vi "Autonomous Independent.vi"   [LabVIEW 2015]
doc: "This VI is called when autonomous begins, and will automatically be terminated when autonomous ends. You can carry out timed or sensor driven robot movement independently without needing to return to the caller."
uses:
  Auton Control.ctl
  <vilib>/Rock Robotics/WPI/Utilities/WPI_GetSetVariantRefNum.vi
  <vilib>/Rock Robotics/Network Tables/NT Read Numeric Array.vi
  <vilib>/Rock Robotics/Network Tables/NT Write Number.vi
  <vilib>/Rock Robotics/Network Tables/NT Write Boolean.vi
  <vilib>/Rock Robotics/Network Tables/NT Write Numeric Array.vi
  navX Library v2/navX Library v2.lvlib
panel:
  # "Be sure to right-click and choose Data Operations>>Make Current Value default if you want to save the array values with the VI"
types:
  T1 = typedef "Auton Control.ctl" = enum16{"Rough Terrain", "Moat", "Ramparts", "Portcullis", "Cheval de Frise", "Rock Wall", "SolenoidControl", "AllStop", "BackOff", "Feeder", "LowBar", "GyroReset", "Shoot", "Scan", "Long Pause", "Short Pause", "Initialize", "Stop", "Straight Forward", "Straight Back", "90 Right", "90 Left", "60 Right", "60 Left"}
  T2 = typedef "WPI_RobotDriveDevRef.ctl" = cluster{"DevStatus":errorcluster, "Motors[]":T3[], "Square Inputs":bool, "Max Output":dbl}
  T3 = typedef "WPI_MotorControlDeviceRef.ctl" = cluster{"DeviceStatus":errorcluster, "Type":T4, "PWM":cluster{"PWM Channel":T5, "DeadBand":T6}, "CAN":cluster{"Device Number":u8, "Control Mode":T7, "Semaphore":T8, "Max Vout":dbl, "TalonSRX Control Mode":T9}, "Invert":bool}
  T4 = typedef "WPI_MotorControlType.ctl" = enum16{"PWM", "CAN", "CANTalonSRX"}
  T5 = typedef "FPGA_DIOPWMChannel.ctl" = enum8{"PWM 0", "PWM 1", "PWM 2", "PWM 3", "PWM 4", "PWM 5", "PWM 6", "PWM 7", "PWM 8", "PWM 9", "PWM MXP 0", "PWM MXP 1", "PWM MXP 2", "PWM MXP 3", "PWM MXP 4", "PWM MXP 5", "PWM MXP 6", "PWM MXP 7", "PWM MXP 8", "PWM MXP 9", "Invalid"}
  T6 = typedef "WPI_PWMDeadband.ctl" = cluster{"Name":string, "maxPositivePwm":i32, "minPositivePwm":i32, "centerPwm":i32, "maxNegativePwm":i32, "minNegativePwm":i32, "angularRange":u16}
  T7 = typedef "WPI_CANJaguar_ControlMode.ctl" = enum8{"Percent VBus", "Current", "Speed", "Position", "Voltage"}
  T8 = typedef "Semaphore RefNum" = refnum<k1>
  T9 = typedef "WPI_CANTalonSRX_APIControlMode.ctl" = enum8{"Percent VBus", "Speed", "Position", "Slave", "Unchanged / Invalid", "Voltage Compensation", "Current", "Motion Profile"}
  T10 = typedef "navX Library v2.lvlib/Z900_navX_DeviceTypeDef.ctl" = cluster{"Interface":cluster{"Protocol":T11, "Update Rate (4Hz-60Hz)":u8, "navX Open TypeDef":variant}, "Notify Packet":refnum<notifier>, "Loop VI Refnum":refnum<vi>, "Ready to Close Occurrence Refnum":refnum<k4>}
  T11 = typedef "navX Library v2.lvlib/Z900_navX_ProtocolTypeDef.ctl" = enum16{"SERIAL", "I2C", "SPI"}
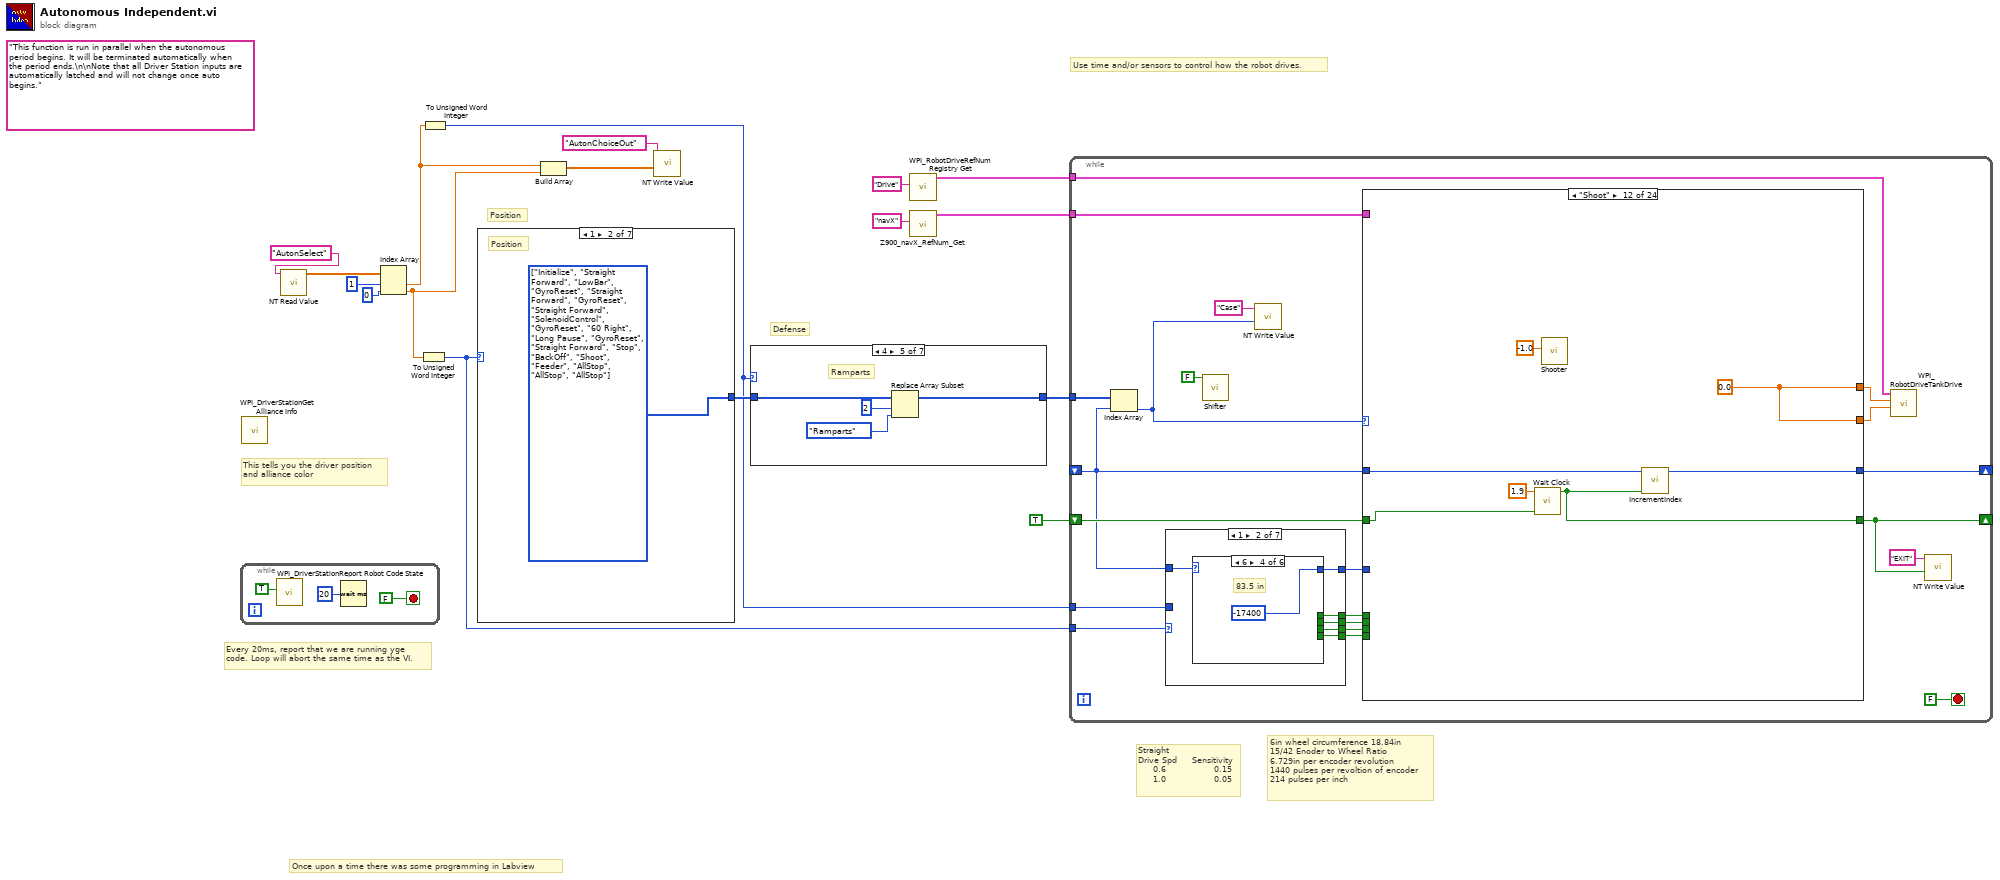
[diagram p0: block diagram]
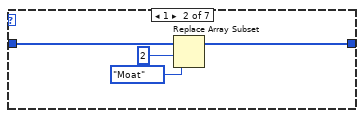
[diagram p3: hidden frame]
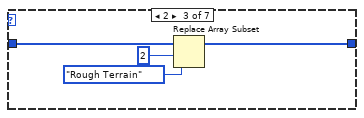
[diagram p4: hidden frame]
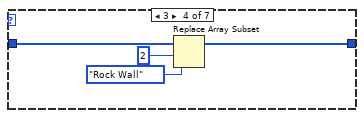
[diagram p5: hidden frame]
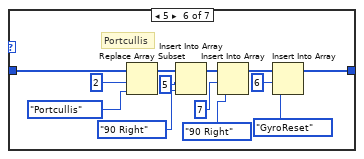
[diagram p6: hidden frame]
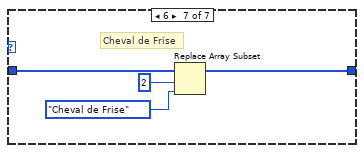
[diagram p7: hidden frame]
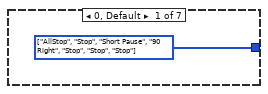
[diagram p8: hidden frame]
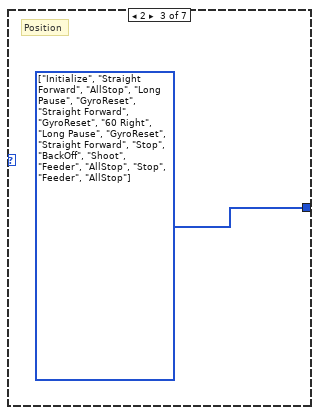
[diagram p9: hidden frame]
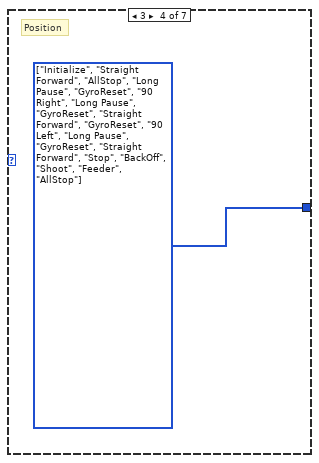
[diagram p10: hidden frame]
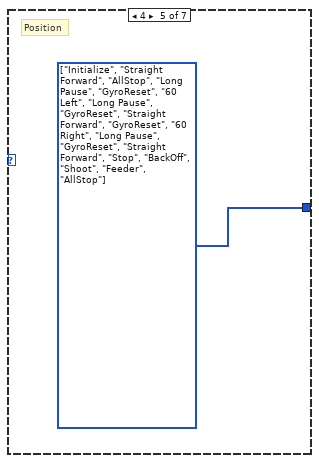
[diagram p11: hidden frame]
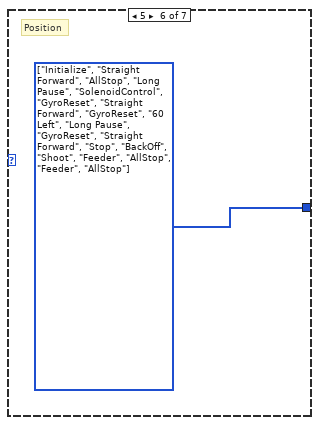
[diagram p12: hidden frame]
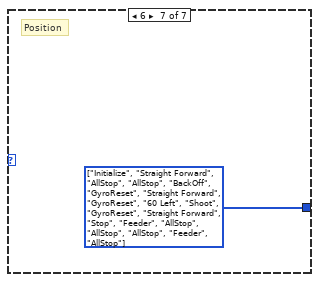
[diagram p13: hidden frame]
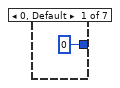
[diagram p14: hidden frame]
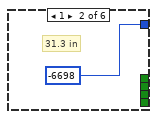
[diagram p16: hidden frame]
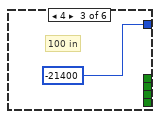
[diagram p17: hidden frame]
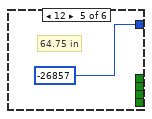
[diagram p18: hidden frame]
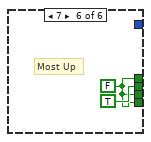
[diagram p19: hidden frame]
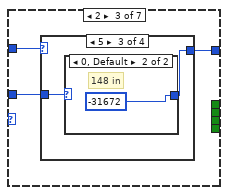
[diagram p20: hidden frame]
diagram:
  (unwired) "This function is run in parallel when the autonomous period begins. It will be terminated automatically when the period ends.\n\nNote that all Driver Station inputs are automatically latched and will not change once auto begins."
  # "Straight\nDrive Spd     Sensitivity\n     0.6                0.15\n     1.0                0.05"
  # "6in wheel circumference 18.84in\n15/42 Enoder to Wheel Ratio\n6.729in per encoder revolution\n1440 pulses per revoltion of encoder\n214 pulses per inch"
  # "Defense"
  # "Position"
  # "Once upon a time there was some programming in Labview"
  # "Every 20ms, report that we are running yge\ncode. Loop will abort the same time as the VI."
  # "Use time and/or sensors to control how the robot drives."
  # "This tells you the driver position\nand alliance color"
  n1 = while {
    stop <- FALSE stop-if-true
    n2 = call <vilib>:"WPI_DriverStationReport Robot Code State.vi"("Autonomous"=TRUE) -> ()  [unwired: 10 in, 1 out]
    n3 = Wait (ms)(milliseconds to wait=u32 20) -> ()  [unwired: 1 out]
  }
  n4 = call <vilib>:"WPI_DriverStationGet Alliance Info.vi"() -> ()  [unwired: 12 out]
  n5 = call-poly <vilib>:"NT Read Value.vi"("Name"="AutonSelect") -> ("Numeric Array"=w9:dbl[])  [unwired: 9 in, 1 out]
  n6 = Index Array(array=w9, index #1=1 ("index"), index #2=0 ("index")) -> (element #1=w2:dbl, element #2=w1:dbl)
  n7 = To Unsigned Word Integer(number=w1) -> (unsigned 16bit integer=w5:u16)
  n8 = To Unsigned Word Integer(number=w2) -> (unsigned 16bit integer=w6:u16)
  n9 = case shown="1" w5 {
    tunnel: [w21 w22 w23 w24 w25 w26 w27] -> w11
    frame 0, Default {
      w21 = T1[] [enum."AllStop", enum."Stop", enum."Short Pause", enum."90 Right", enum."Stop", enum."Stop", enum."Stop"] items=["Rough Terrain", "Moat", "Ramparts", "Portcullis", "Cheval de Frise", "Rock Wall", "SolenoidControl", "AllStop", "BackOff", "Feeder", "LowBar", "GyroReset", "Shoot", "Scan", "Long Pause", "Short Pause", "Initialize", "Stop", "Straight Forward", "Straight Back", "90 Right", "90 Left", "60 Right", "60 Left"] ("Array")
    }
    frame 1 {
      w22 = T1[] [enum."Initialize", enum."Straight Forward", enum."LowBar", enum."GyroReset", enum."Straight Forward", enum."GyroReset", enum."Straight Forward", enum."SolenoidControl", enum."GyroReset", enum."60 Right", enum."Long Pause", enum."GyroReset", enum."Straight Forward", enum."Stop", enum."BackOff", enum."Shoot", enum."Feeder", enum."AllStop", enum."AllStop", enum."AllStop"] items=["Rough Terrain", "Moat", "Ramparts", "Portcullis", "Cheval de Frise", "Rock Wall", "SolenoidControl", "AllStop", "BackOff", "Feeder", "LowBar", "GyroReset", "Shoot", "Scan", "Long Pause", "Short Pause", "Initialize", "Stop", "Straight Forward", "Straight Back", "90 Right", "90 Left", "60 Right", "60 Left"] ("Array")
      # "Position"
    }
    frame 2 {
      w23 = T1[] [enum."Initialize", enum."Straight Forward", enum."AllStop", enum."Long Pause", enum."GyroReset", enum."Straight Forward", enum."GyroReset", enum."60 Right", enum."Long Pause", enum."GyroReset", enum."Straight Forward", enum."Stop", enum."BackOff", enum."Shoot", enum."Feeder", enum."AllStop", enum."Stop", enum."Feeder", enum."AllStop"] items=["Rough Terrain", "Moat", "Ramparts", "Portcullis", "Cheval de Frise", "Rock Wall", "SolenoidControl", "AllStop", "BackOff", "Feeder", "LowBar", "GyroReset", "Shoot", "Scan", "Long Pause", "Short Pause", "Initialize", "Stop", "Straight Forward", "Straight Back", "90 Right", "90 Left", "60 Right", "60 Left"] ("Array")
      # "Position"
    }
    frame 3 {
      w24 = T1[] [enum."Initialize", enum."Straight Forward", enum."AllStop", enum."Long Pause", enum."GyroReset", enum."90 Right", enum."Long Pause", enum."GyroReset", enum."Straight Forward", enum."GyroReset", enum."90 Left", enum."Long Pause", enum."GyroReset", enum."Straight Forward", enum."Stop", enum."BackOff", enum."Shoot", enum."Feeder", enum."AllStop"] items=["Rough Terrain", "Moat", "Ramparts", "Portcullis", "Cheval de Frise", "Rock Wall", "SolenoidControl", "AllStop", "BackOff", "Feeder", "LowBar", "GyroReset", "Shoot", "Scan", "Long Pause", "Short Pause", "Initialize", "Stop", "Straight Forward", "Straight Back", "90 Right", "90 Left", "60 Right", "60 Left"] ("Array")
      # "Position"
    }
    frame 4 {
      w25 = T1[] [enum."Initialize", enum."Straight Forward", enum."AllStop", enum."Long Pause", enum."GyroReset", enum."60 Left", enum."Long Pause", enum."GyroReset", enum."Straight Forward", enum."GyroReset", enum."60 Right", enum."Long Pause", enum."GyroReset", enum."Straight Forward", enum."Stop", enum."BackOff", enum."Shoot", enum."Feeder", enum."AllStop"] items=["Rough Terrain", "Moat", "Ramparts", "Portcullis", "Cheval de Frise", "Rock Wall", "SolenoidControl", "AllStop", "BackOff", "Feeder", "LowBar", "GyroReset", "Shoot", "Scan", "Long Pause", "Short Pause", "Initialize", "Stop", "Straight Forward", "Straight Back", "90 Right", "90 Left", "60 Right", "60 Left"] ("Array")
      # "Position"
    }
    frame 5 {
      w26 = T1[] [enum."Initialize", enum."Straight Forward", enum."AllStop", enum."Long Pause", enum."SolenoidControl", enum."GyroReset", enum."Straight Forward", enum."GyroReset", enum."60 Left", enum."Long Pause", enum."GyroReset", enum."Straight Forward", enum."Stop", enum."BackOff", enum."Shoot", enum."Feeder", enum."AllStop", enum."Feeder", enum."AllStop"] items=["Rough Terrain", "Moat", "Ramparts", "Portcullis", "Cheval de Frise", "Rock Wall", "SolenoidControl", "AllStop", "BackOff", "Feeder", "LowBar", "GyroReset", "Shoot", "Scan", "Long Pause", "Short Pause", "Initialize", "Stop", "Straight Forward", "Straight Back", "90 Right", "90 Left", "60 Right", "60 Left"] ("Array")
      # "Position"
    }
    frame 6 {
      w27 = T1[] [enum."Initialize", enum."Straight Forward", enum."AllStop", enum."AllStop", enum."BackOff", enum."GyroReset", enum."Straight Forward", enum."GyroReset", enum."60 Left", enum."Shoot", enum."GyroReset", enum."Straight Forward", enum."Stop", enum."Feeder", enum."AllStop", enum."AllStop", enum."AllStop", enum."Feeder", enum."AllStop"] items=["Rough Terrain", "Moat", "Ramparts", "Portcullis", "Cheval de Frise", "Rock Wall", "SolenoidControl", "AllStop", "BackOff", "Feeder", "LowBar", "GyroReset", "Shoot", "Scan", "Long Pause", "Short Pause", "Initialize", "Stop", "Straight Forward", "Straight Back", "90 Right", "90 Left", "60 Right", "60 Left"] ("Array")
      # "Position"
    }
  }
  n10 = Build Array(w2, w1) -> (w3:dbl[])
  n11 = call-poly <vilib>:"NT Write Value.vi"("Numeric Array"=w3, "Name"="AutonChoiceOut") -> ()  [unwired: 9 in, 1 out]
  n12 = case shown="4" w6 {
    tunnel: w11 -> [w28 w32 w36 w40 w44 w57 w61]
    tunnel: [w28 w31 w35 w39 w43 w47 w60] -> w10
    frame 0, Default {
      # "Low Bar"
    }
    frame 1 {
      n13 = Replace Array Subset(array=w32, new element=Auton_Control."Moat" ("new element/subarray"), index=2) -> (w31:T1[])
    }
    frame 2 {
      n14 = Replace Array Subset(array=w36, new element=Auton_Control."Rough Terrain" ("new element/subarray"), index=2) -> (w35:T1[])
    }
    frame 3 {
      n15 = Replace Array Subset(array=w40, new element=Auton_Control."Rock Wall" ("new element/subarray"), index=2) -> (w39:T1[])
    }
    frame 4 {
      # "Ramparts"
      n16 = Replace Array Subset(array=w44, new element=Auton_Control."Ramparts" ("new element/subarray"), index=2) -> (w43:T1[])
    }
    frame 5 {
      # "Portcullis"
      n17 = Replace Array Subset(array=w57, new element=Auton_Control."Portcullis" ("new element/subarray"), index=2) -> (w54:T1[])
      n18 = Insert Into Array(array=w54, index=5, new element=Auton_Control."90 Right" ("new element/subarray")) -> (w51:T1[])
      n19 = Insert Into Array(array=w51, index=7, new element=Auton_Control."90 Right" ("new element/subarray")) -> (w48:T1[])
      n20 = Insert Into Array(array=w48, index=6, new element=Auton_Control."GyroReset" ("new element/subarray")) -> (w47:T1[])
    }
    frame 6 {
      # "Cheval de Frise"
      n21 = Replace Array Subset(array=w61, new element=Auton_Control."Cheval de Frise" ("new element/subarray"), index=2) -> (w60:T1[])
    }
  }
  n22 = call <vilib>:"WPI_RobotDriveRefNum Registry Get.vi"("refnum name"="Drive") -> ("RobotDriveDevRef"=w14:T2)  [unwired: 9 in, 1 out]
  n23 = call "Z900_navX_RefNum_Get.vi"("refnum name"="navX") -> ("navX Device"=w17:T10)  [unwired: 9 in, 1 out]
  n24 = while {
    shift-right: [w69] -> _
    shift-left: _ -> [w72]
    shift-right: [w64] -> _
    shift-left: TRUE -> [w82]
    tunnel: w17 -> [w77]
    tunnel: w14 -> [w74]
    tunnel: w10 -> [w73]
    tunnel: w5 -> [w70]
    tunnel: w6 -> [w63]
    stop <- FALSE stop-if-true
    n25 = Index Array(array=w73, index=w72) -> (element=w79:T1)
    n26 = case shown="1" w70 {
      tunnel: w72 -> [_ w89 w98 w107 w116 w129 w139]
      tunnel: [0 w88 w97 w106 w115 w128 w138] -> w71
      tunnel: [_ w87 _ _ _ w125 _] -> w68
      tunnel: [_ w86 _ _ _ w124 _] -> w67
      tunnel: [_ w85 _ _ _ w123 _] -> w66
      tunnel: [_ w84 _ _ _ w126 _] -> w65
      tunnel: w63 -> [_ _ w96 w105 w114 w127 _]
      frame 0, Default {
      }
      frame 1 {
        n27 = case shown="6" w89 {
          tunnel: [_ -6698 -21400 -17400 -26857 _] -> w88
          tunnel: [_ _ _ _ _ w94] -> w87
          tunnel: [_ _ _ _ _ TRUE] -> w86
          tunnel: [_ _ _ _ _ w94] -> w85
          tunnel: [_ _ _ _ _ w94] -> w84
          frame 0, Default {
          }
          frame 1 {
            # "31.3 in"
          }
          frame 4 {
            # "100 in"
          }
          frame 6 {
            # "83.5 in"
          }
          frame 12 {
            # "64.75 in"
          }
          frame 7 {
            w94 = FALSE
            # "Most Up"
          }
        }
      }
      frame 2 {
        n28 = case shown="5" w98 {
          tunnel: [_ -6698 w101 -13500] -> w97
          tunnel: w96 -> [_ _ w100 _]
          frame 0, Default {
          }
          frame 1 {
            # "31.3 in"
          }
          frame 5 {
            n29 = case shown="0, Default" w100 {
              tunnel: [-2500 -31672] -> w101
              frame 5 {
                # "10.56 in"
              }
              frame 0, Default {
                # "148 in"
              }
            }
          }
          frame 10 {
            # "62.3 in"
          }
        }
      }
      frame 3 {
        n30 = case shown="8" w107 {
          tunnel: [_ -6698 w110 -33000] -> w106
          tunnel: w105 -> [_ _ w109 _]
          frame 0, Default {
          }
          frame 1 {
            # "31.3 in"
          }
          frame 8 {
            n31 = case shown="0, Default" w109 {
              tunnel: [-6869 -7960] -> w110
              frame 5 {
              }
              frame 0, Default {
                # "38.2 in"
              }
            }
          }
          frame 13 {
            # "154"
          }
        }
      }
      frame 4 {
        n32 = case shown="8" w116 {
          tunnel: [_ -6698 w119 -34850] -> w115
          tunnel: w114 -> [_ _ w118 _]
          frame 0, Default {
          }
          frame 1 {
            # "31.3 in"
          }
          frame 8 {
            n33 = case shown="5" w118 {
              tunnel: [-3659 -8945] -> w119
              frame 0, Default {
                # "17.1 in"
              }
              frame 5 {
              }
            }
          }
          frame 13 {
            # "161.8 in"
          }
        }
      }
      frame 5 {
        n34 = case shown="6" w129 {
          tunnel: [_ -6698 _ w134 -12100] -> w128
          tunnel: w127 -> [_ _ _ w133 _]
          tunnel: [_ _ TRUE _ _] -> w126
          tunnel: [_ _ w131 _ _] -> w125
          tunnel: [_ _ w131 _ _] -> w124
          tunnel: [_ _ w131 _ _] -> w123
          frame 0, Default {
          }
          frame 1 {
            # "31.3 in"
          }
          frame 4 {
            w131 = FALSE
            # "All Up"
          }
          frame 6 {
            n35 = case shown="0, Default" w133 {
              tunnel: [-28700 -27451] -> w134
              frame 0, Default {
                # "134"
              }
              frame 5 {
              }
            }
          }
          frame 11 {
            # "55.7 in"
          }
        }
      }
      frame 6 {
        n36 = case shown="1" w139 {
          tunnel: [_ -6698] -> w138
          frame 0, Default {
          }
          frame 1 {
            # "31.3 in"
          }
        }
      }
    }
    n37 = call "Shifter.vi"("Shift"=FALSE) -> ()  [unwired: 11 in]
    n38 = call-poly <vilib>:"NT Write Value.vi"("Numeric"=w79, "Name"="Case") -> ()  [unwired: 9 in, 1 out]
    n39 = case shown="\"Shoot\"" w79 {
      tunnel: [w144 w145 w161 w182 w191 w223 w245 w260 w262 w268 w273 w281 w289 0.0 ("Left") w305 w317 w323 w333 w345 w407 w469 w520 w581 w644] -> w76
      tunnel: [w144 w146 w160 w183 w190 w222 w244 w260 w262 w268 w273 w281 w289 0.0 ("Left") w306 w317 w323 w333 w346 w408 w470 w521 w582 w645] -> w75
      tunnel: w82 -> [w141 w153 w168 w186 w201 w216 w238 w249 w264 w270 w274 w279 w290 w296 w307 w313 w321 w326 w335 w397 w459 w523 w574 w647]
      tunnel: w72 -> [w143 w152 w167 w189 w204 w225 w247 w257 w265 w271 w276 w283 w292 w298 w311 w319 w322 w328 w337 w399 w461 w525 w576 w643]
      tunnel: w77 -> [_ w154 w169 w185 w200 w219 w241 w255 _ _ _ _ w287 _ _ _ _ _ w350 w412 w474 w536 w580 _]
      tunnel: w71 -> [_ _ _ _ _ w206 w228 _ _ _ _ _ _ _ _ _ _ _ _ _ _ _ _ _]
      tunnel: [w142 w150 w165 w188 w203 w224 w246 w256 w266 w272 w275 w282 w291 w297 w310 w318 w322 w327 w336 w398 w460 w524 w575 w642] -> w69
      tunnel: w68 -> [_ _ _ _ _ _ _ _ _ _ _ _ _ _ _ _ _ w332 _ _ _ _ _ _]
      tunnel: w67 -> [_ _ _ _ _ _ _ _ _ _ _ _ _ _ _ _ _ w331 _ _ _ _ _ _]
      tunnel: w66 -> [_ _ _ _ _ _ _ _ _ _ _ _ _ _ _ _ _ w330 _ _ _ _ _ _]
      tunnel: w65 -> [_ _ _ _ _ _ _ _ _ _ _ _ _ _ _ _ _ w329 _ _ _ _ _ _]
      tunnel: [w141 w151 w166 w184 w199 w207 w229 w250 w261 w267 w274 w278 w284 w296 w308 w312 w321 w324 w334 w396 w458 w522 w579 w641] -> w64
      frame "Stop", Default {
        w144 = 0.0
        n40 = call "IncrementIndex.vi"("Increment?"=w141, "IndexIn"=w143) -> ("IndexOut"=w142:i32)  [unwired: 9 in]
      }
      frame "90 Right" {
        w148 = 0.55  # Min Power
        w149 = 0.5  # Target Range
        w157 = 90.0  # Target Position
        w158 = 55.0  # Slow Range
        w159 = 1.0  # Motor Power In
        # "Target position"
        n41 = call "GyroActions.vi"("Zero"=FALSE, "Update"=FALSE, "navX Device"=w154) -> ("Yaw"=w156:dbl)  [unwired: 4 in, 4 out]
        n42 = call "TurnSmooth.vi"("Min Power"=w148, "First Time?"=w153, "Target Range"=w149, "Current Position"=w156, "Target Position"=w157, "Slow Range"=w158, "Motor Power In"=w159) -> ("Done"=w151:bool, "Motor Power Out"=w145:dbl)  [unwired: 3 in]
        n43 = call "IncrementIndex.vi"("Increment?"=w151, "IndexIn"=w152) -> ("IndexOut"=w150:i32)  [unwired: 9 in]
        n44 = Negate(x=w145) -> (-x=w146:dbl)
      }
      frame "90 Left" {
        w163 = 0.55  # Min Power
        w164 = 0.5  # Target Range
        w172 = -90.0  # Target Position
        w173 = 55.0  # Slow Range
        w174 = 1.0  # Motor Power In
        # "Target position"
        n45 = call "GyroActions.vi"("Zero"=FALSE, "Update"=FALSE, "navX Device"=w169) -> ("Yaw"=w171:dbl)  [unwired: 4 in, 4 out]
        n46 = call "TurnSmooth.vi"("Min Power"=w163, "First Time?"=w168, "Target Range"=w164, "Current Position"=w171, "Target Position"=w172, "Slow Range"=w173, "Motor Power In"=w174) -> ("Done"=w166:bool, "Motor Power Out"=w160:dbl)  [unwired: 3 in]
        n47 = Negate(x=w160) -> (-x=w161:dbl)
        n48 = call "IncrementIndex.vi"("Increment?"=w166, "IndexIn"=w167) -> ("IndexOut"=w165:i32)  [unwired: 9 in]
      }
      frame "60 Right" {
        w176 = 0.65  # Min Power
        w177 = 0.5  # Target Range
        w178 = 60.0  # Target Position
        w179 = 30.0  # Slow Range
        w180 = 0.9  # Motor Power In
        n49 = call "GyroActions.vi"("Zero"=FALSE, "Update"=FALSE, "navX Device"=w185) -> ("Yaw"=w181:dbl)  [unwired: 4 in, 4 out]
        n50 = call "TurnSmooth.vi"("Min Power"=w176, "First Time?"=w186, "Target Range"=w177, "Current Position"=w181, "Target Position"=w178, "Slow Range"=w179, "Motor Power In"=w180) -> ("Done"=w184:bool, "Motor Power Out"=w182:dbl)  [unwired: 3 in]
        n51 = call "IncrementIndex.vi"("Increment?"=w184, "IndexIn"=w189) -> ("IndexOut"=w188:i32)  [unwired: 9 in]
        n52 = Negate(x=w182) -> (-x=w183:dbl)
      }
      frame "60 Left" {
        w193 = 0.6  # Min Power
        w194 = 0.5  # Target Range
        w195 = -60.0  # Target Position
        w196 = 30.0  # Slow Range
        w197 = 0.9  # Motor Power In
        n53 = call "GyroActions.vi"("Zero"=FALSE, "Update"=FALSE, "navX Device"=w200) -> ("Yaw"=w198:dbl)  [unwired: 4 in, 4 out]
        n54 = call "TurnSmooth.vi"("Min Power"=w193, "First Time?"=w201, "Target Range"=w194, "Current Position"=w198, "Target Position"=w195, "Slow Range"=w196, "Motor Power In"=w197) -> ("Done"=w199:bool, "Motor Power Out"=w190:dbl)  [unwired: 3 in]
        n55 = call "IncrementIndex.vi"("Increment?"=w199, "IndexIn"=w204) -> ("IndexOut"=w203:i32)  [unwired: 9 in]
        n56 = Negate(x=w190) -> (-x=w191:dbl)
      }
      frame "Straight Forward" {
        w220 = 0.25  # Range
        w221 = -1.0  # Motor Speed
        n57 = call "GyroActions.vi"("Zero"=FALSE, "Update"=FALSE, "navX Device"=w219) -> ("Yaw"=w214:dbl)  [unwired: 4 in, 4 out]
        n58 = call "Wait Clock.vi"("First Time?"=w216, "Target Time"=5.0) -> ("Completed"=w210:bool)  [unwired: 9 in]
        n59 = call "EncoderLeftDrive.vi"() -> ("Position_out"=w212:i32)  [unwired: 11 in]
        n60 = call "EncoderRightDrive.vi"() -> ("Position_out"=w211:i32)  [unwired: 11 in]
        n61 = Less Or Equal?(x=w212, y=w206) -> (x <= y?=w209:bool)
        n62 = Less Or Equal?(x=w211, y=w206) -> (x <= y?=w208:bool)
        n63 = Not(x=w216) -> (.not. x?=w217:bool)
        n64 = Compound Arithmetic op=OR(w210, w209, w208) -> (w207:bool)
        n65 = call "LockedHeading.vi"("LockHeading"=w217, "Heading In"=w214) -> ("LockedHeading"=w215:dbl)  [unwired: 9 in]
        n66 = call "DriveStraight.vi"("Sensitivity"=0.05, "Range"=w220, "Motor Speed"=w221, "Target"=w215, "Yaw"=w214) -> ("Right"=w223:dbl, "Left"=w222:dbl)  [unwired: 5 in]
        n67 = call "IncrementIndex.vi"("Increment?"=w207, "IndexIn"=w225) -> ("IndexOut"=w224:i32)  [unwired: 9 in]
      }
      frame "Straight Back" {
        w242 = 0.25  # Range
        w243 = 1.0  # Motor Speed
        n68 = call "GyroActions.vi"("Zero"=FALSE, "Update"=FALSE, "navX Device"=w241) -> ("Yaw"=w236:dbl)  [unwired: 4 in, 4 out]
        n69 = call "Wait Clock.vi"("First Time?"=w238, "Target Time"=5.0) -> ("Completed"=w232:bool)  [unwired: 9 in]
        n70 = call "EncoderLeftDrive.vi"() -> ("Position_out"=w234:i32)  [unwired: 11 in]
        n71 = call "EncoderRightDrive.vi"() -> ("Position_out"=w233:i32)  [unwired: 11 in]
        n72 = Greater Or Equal?(x=w234, y=w228) -> (x >= y?=w231:bool)
        n73 = Greater Or Equal?(x=w233, y=w228) -> (x >= y?=w230:bool)
        n74 = Not(x=w238) -> (.not. x?=w239:bool)
        n75 = Compound Arithmetic op=OR(w232, w231, w230) -> (w229:bool)
        n76 = call "LockedHeading.vi"("LockHeading"=w239, "Heading In"=w236) -> ("LockedHeading"=w237:dbl)  [unwired: 9 in]
        n77 = call "DriveStraight.vi"("Sensitivity"=0.05, "Range"=w242, "Motor Speed"=w243, "Target"=w237, "Yaw"=w236) -> ("Right"=w245:dbl, "Left"=w244:dbl)  [unwired: 5 in]
        n78 = call "IncrementIndex.vi"("Increment?"=w229, "IndexIn"=w247) -> ("IndexOut"=w246:i32)  [unwired: 9 in]
      }
      frame "Initialize" {
        w260 = 0.0
        n79 = call "EncoderLeftDrive.vi"("Zero"=TRUE) -> ()  [unwired: 10 in, 1 out]
        n80 = call "GyroActions.vi"("Zero"=w249, "Update"=FALSE, "navX Device"=w255) -> ("Yaw"=w251:dbl)  [unwired: 4 in, 4 out]
        n81 = call "EncoderRightDrive.vi"("Zero"=TRUE) -> ()  [unwired: 10 in, 1 out]
        n82 = In Range and Coerce(upper limit=0.5, x=w251, lower limit=-0.5) -> (In Range?=w250:bool)  [unwired: 1 out]
        n83 = call "IncrementIndex.vi"("Increment?"=w250, "IndexIn"=w257) -> ("IndexOut"=w256:i32)  [unwired: 9 in]
        n84 = call "2Slnd.vi"() -> ()  [unwired: 12 in]
      }
      frame "Short Pause" {
        w262 = 0.0 ("Left")
        n85 = call "Wait Clock.vi"("First Time?"=w264, "Target Time"=0.1) -> ("Completed"=w261:bool)  [unwired: 9 in]
        n86 = call "IncrementIndex.vi"("Increment?"=w261, "IndexIn"=w265) -> ("IndexOut"=w266:i32)  [unwired: 9 in]
      }
      frame "Long Pause" {
        w268 = 0.0 ("Left")
        n87 = call "Wait Clock.vi"("First Time?"=w270, "Target Time"=0.5) -> ("Completed"=w267:bool)  [unwired: 9 in]
        n88 = call "IncrementIndex.vi"("Increment?"=w267, "IndexIn"=w271) -> ("IndexOut"=w272:i32)  [unwired: 9 in]
      }
      frame "Scan" {
        w273 = 0.0 ("Left")
        n89 = call "IncrementIndex.vi"("Increment?"=w274, "IndexIn"=w276) -> ("IndexOut"=w275:i32)  [unwired: 9 in]
      }
      frame "Shoot" {
        w281 = 0.0 ("Left")
        n90 = call "Wait Clock.vi"("First Time?"=w279, "Target Time"=1.9) -> ("Completed"=w278:bool)  [unwired: 9 in]
        n91 = call "Shooter.vi"("Power"=-1.0) -> ()  [unwired: 11 in]
        n92 = call "IncrementIndex.vi"("Increment?"=w278, "IndexIn"=w283) -> ("IndexOut"=w282:i32)  [unwired: 9 in]
      }
      frame "GyroReset" {
        w289 = 0.0 ("Left")
        n93 = call "GyroActions.vi"("Zero"=w290, "Update"=FALSE, "navX Device"=w287) -> ("Yaw"=w293:dbl)  [unwired: 4 in, 4 out]
        n94 = call "EncoderLeftDrive.vi"("Zero"=TRUE) -> ()  [unwired: 10 in, 1 out]
        n95 = call "EncoderRightDrive.vi"("Zero"=TRUE) -> ()  [unwired: 10 in, 1 out]
        n96 = In Range and Coerce(upper limit=0.5, x=w293, lower limit=-0.5) -> (In Range?=w284:bool)  [unwired: 1 out]
        n97 = call "IncrementIndex.vi"("Increment?"=w284, "IndexIn"=w292) -> ("IndexOut"=w291:i32)  [unwired: 9 in]
      }
      frame "LowBar" {
        w299 = FALSE ("MostDown")
        n98 = call "IncrementIndex.vi"("Increment?"=w296, "IndexIn"=w298) -> ("IndexOut"=w297:i32)  [unwired: 9 in]
        n99 = call "2Slnd.vi"("AllUp"=w299, "AllDown"=w296, "MostUp"=w299, "MostDown"=w299) -> ()  [unwired: 8 in]
      }
      frame "Feeder" {
        n100 = call "Wait Clock.vi"("First Time?"=w307, "Target Time"=2.0) -> ("Completed"=w308:bool)  [unwired: 9 in]
        n101 = call "Shooter.vi"("Power"=-1.0) -> ()  [unwired: 11 in]
        n102 = call "IncrementIndex.vi"("Increment?"=w308, "IndexIn"=w311) -> ("IndexOut"=w310:i32)  [unwired: 9 in]
        n103 = call "Feeder.vi"("Power"=1.0) -> ()  [unwired: 11 in]
        n104 = call "AllOff.vi"("ButtonIn"=w307) -> ("RightOut"=w305:dbl, "LeftOut"=w306:dbl, "WandOut"=w304:dbl)  [unwired: 7 in, 1 out]
        n105 = call "Wand.vi"("Power"=w304) -> ()  [unwired: 11 in]
      }
      frame "BackOff" {
        w317 = 0.0 ("LeftOut")
        n106 = call "PhotoeyeOut.vi"("MotorPower"=-0.2, "Button"=w313, "MotorIn"=0.0) -> ("Complete"=w312:bool, "MotorOut"=w316:dbl)  [unwired: 7 in]
        n107 = call "Feeder.vi"("Power"=w316) -> ()  [unwired: 11 in]
        n108 = call "IncrementIndex.vi"("Increment?"=w312, "IndexIn"=w319) -> ("IndexOut"=w318:i32)  [unwired: 9 in]
      }
      frame "AllStop" {
        w320 = 0.0 ("Power")
        w323 = 0.0 ("LeftOut")
        n109 = call "Wand.vi"("Power"=w320) -> ()  [unwired: 11 in]
        n110 = call "Shooter.vi"("Power"=w320) -> ()  [unwired: 11 in]
        n111 = call "Feeder.vi"("Power"=w320) -> ()  [unwired: 11 in]
      }
      frame "SolenoidControl" {
        w333 = 0.0 ("LeftOut")
        n112 = call "2Slnd.vi"("AllUp"=w329, "AllDown"=w330, "MostUp"=w331, "MostDown"=w332) -> ()  [unwired: 8 in]
        n113 = call "Wait Clock.vi"("First Time?"=w326, "Target Time"=0.5) -> ("Completed"=w324:bool)  [unwired: 9 in]
        n114 = call "IncrementIndex.vi"("Increment?"=w324, "IndexIn"=w328) -> ("IndexOut"=w327:i32)  [unwired: 9 in]
      }
      frame "Rock Wall" {
        n115 = call "GyroActions.vi"("navX Device"=w350) -> ("Pitch"=w341:dbl, "Yaw"=w339:dbl, "Roll"=w340:dbl)  [unwired: 6 in, 2 out]
        n116 = Not(x=w335) -> (.not. x?=w349:bool)
        n117 = call "LockedHeading.vi"("LockHeading"=w349, "Heading In"=w339) -> ("LockedHeading"=w338:dbl)  [unwired: 9 in]
        n118 = call "DriveStraight.vi"("Sensitivity"=0.05, "Range"=0.25, "Motor Speed"=-1.0, "Target"=w338, "Yaw"=w339) -> ("Right"=w347:dbl, "Left"=w348:dbl)  [unwired: 5 in]
        n119 = disable-structure shown="Enabled" {
          disable-tunnel: w348 -> [w370 w395]
          disable-tunnel: w347 -> [w369 w394]
          disable-tunnel: [w366 w395] -> w346
          disable-tunnel: [w365 w394] -> w345
          disable-tunnel: w341 -> [w364 _]
          disable-tunnel: w340 -> [w363 _]
          disable-tunnel: w339 -> [w362 _]
          disable-tunnel: w338 -> [w361 _]
          disable-tunnel: w335 -> [w360 w393]
          disable-tunnel: [w359 w391] -> w334
          frame Disabled {
            n120 = call "DefenseCrosser.vi"("FirstTime?"=w360, "Wait Time"=1.0, "Roll"=w363, "Pitch"=w364, "RightIn"=w369, "LeftIn"=w370) -> ("Complete?"=w356:bool, "RightOut"=w367:dbl, "LeftOut"=w368:dbl)  [unwired: 3 in]
            n121 = feedback #1(FALSE) -> (w354:bool)
            n122 = Select(t=TRUE, s=w356, f=w354) -> (s? t:f=w352:bool)
            n123 = feedback-in #1(w352) -> ()
            n124 = case shown="True" w352 {
              selector: w352 -> [_ w378]
              tunnel: [FALSE w376] -> w357
              frame False {
              }
              frame True {
                n125 = Not(x=w378) -> (.not. x?=w377:bool)
                n126 = feedback-in #2(w377) -> ()
                n127 = feedback #2(TRUE) -> (w376:bool)
              }
            }
            n128 = case shown="True" w352 {
              tunnel: [FALSE ("Completed") w374] -> w358
              tunnel: w357 -> [_ w372]
              frame False {
              }
              frame True {
                n129 = call "Wait Clock.vi"("First Time?"=w372, "Target Time"=1.0) -> ("Completed"=w374:bool)  [unwired: 9 in]
              }
            }
            n130 = case shown="True" w358 {
              tunnel: w368 -> [w381 w390]
              tunnel: w367 -> [w380 w389]
              tunnel: [w381 w388] -> w366
              tunnel: [w380 w387] -> w365
              tunnel: w352 -> [_ w386]
              tunnel: w362 -> [_ w385]
              tunnel: w361 -> [_ w384]
              tunnel: [FALSE ("Complete") w383] -> w359
              frame False {
              }
              frame True {
                n131 = call "Straighten.vi"("Go"=w386, "LockedHeading"=w384, "Yaw"=w385, "RightIn"=w389, "LeftIn"=w390) -> ("Complete"=w383:bool, "RightOut"=w387:dbl, "LeftOut"=w388:dbl)  [unwired: 4 in]
              }
            }
          }
          frame Enabled {
            n132 = call "Wait Clock.vi"("First Time?"=w393, "Target Time"=1.8) -> ("Completed"=w391:bool)  [unwired: 9 in]
          }
        }
        n133 = call "IncrementIndex.vi"("Increment?"=w334, "IndexIn"=w337) -> ("IndexOut"=w336:i32)  [unwired: 9 in]
      }
      frame "Moat" {
        n134 = call "GyroActions.vi"("navX Device"=w412) -> ("Pitch"=w403:dbl, "Yaw"=w401:dbl, "Roll"=w402:dbl)  [unwired: 6 in, 2 out]
        n135 = Not(x=w397) -> (.not. x?=w411:bool)
        n136 = call "LockedHeading.vi"("LockHeading"=w411, "Heading In"=w401) -> ("LockedHeading"=w400:dbl)  [unwired: 9 in]
        n137 = call "DriveStraight.vi"("Sensitivity"=0.05, "Range"=0.25, "Motor Speed"=-1.0, "Target"=w400, "Yaw"=w401) -> ("Right"=w409:dbl, "Left"=w410:dbl)  [unwired: 5 in]
        n138 = disable-structure shown="Enabled" {
          disable-tunnel: w410 -> [w432 w457]
          disable-tunnel: w409 -> [w431 w456]
          disable-tunnel: [w428 w457] -> w408
          disable-tunnel: [w427 w456] -> w407
          disable-tunnel: w403 -> [w426 _]
          disable-tunnel: w402 -> [w425 _]
          disable-tunnel: w401 -> [w424 _]
          disable-tunnel: w400 -> [w423 _]
          disable-tunnel: w397 -> [w422 w455]
          disable-tunnel: [w421 w454] -> w396
          frame Disabled {
            n139 = call "DefenseCrosser.vi"("FirstTime?"=w422, "Wait Time"=1.5, "Roll"=w425, "Pitch"=w426, "RightIn"=w431, "LeftIn"=w432) -> ("Complete?"=w418:bool, "RightOut"=w429:dbl, "LeftOut"=w430:dbl)  [unwired: 3 in]
            n140 = feedback #3(FALSE) -> (w416:bool)
            n141 = Select(t=TRUE, s=w418, f=w416) -> (s? t:f=w414:bool)
            n142 = feedback-in #3(w414) -> ()
            n143 = case shown="True" w414 {
              selector: w414 -> [_ w440]
              tunnel: [FALSE w438] -> w419
              frame False {
              }
              frame True {
                n144 = Not(x=w440) -> (.not. x?=w439:bool)
                n145 = feedback-in #4(w439) -> ()
                n146 = feedback #4(TRUE) -> (w438:bool)
              }
            }
            n147 = case shown="True" w414 {
              tunnel: [FALSE ("Completed") w436] -> w420
              tunnel: w419 -> [_ w434]
              frame False {
              }
              frame True {
                n148 = call "Wait Clock.vi"("First Time?"=w434, "Target Time"=1.0) -> ("Completed"=w436:bool)  [unwired: 9 in]
              }
            }
            n149 = case shown="True" w420 {
              tunnel: w430 -> [w443 w452]
              tunnel: w429 -> [w442 w451]
              tunnel: [w443 w450] -> w428
              tunnel: [w442 w449] -> w427
              tunnel: w414 -> [_ w448]
              tunnel: w424 -> [_ w447]
              tunnel: w423 -> [_ w446]
              tunnel: [FALSE ("Complete") w445] -> w421
              frame False {
              }
              frame True {
                n150 = call "Straighten.vi"("Go"=w448, "LockedHeading"=w446, "Yaw"=w447, "RightIn"=w451, "LeftIn"=w452) -> ("Complete"=w445:bool, "RightOut"=w449:dbl, "LeftOut"=w450:dbl)  [unwired: 4 in]
              }
            }
          }
          frame Enabled {
            n151 = call "Wait Clock.vi"("First Time?"=w455, "Target Time"=2.3) -> ("Completed"=w454:bool)  [unwired: 9 in]
          }
        }
        n152 = call "IncrementIndex.vi"("Increment?"=w396, "IndexIn"=w399) -> ("IndexOut"=w398:i32)  [unwired: 9 in]
      }
      frame "Rough Terrain" {
        n153 = call "GyroActions.vi"("navX Device"=w474) -> ("Pitch"=w465:dbl, "Yaw"=w463:dbl, "Roll"=w464:dbl)  [unwired: 6 in, 2 out]
        n154 = Not(x=w459) -> (.not. x?=w473:bool)
        n155 = call "LockedHeading.vi"("LockHeading"=w473, "Heading In"=w463) -> ("LockedHeading"=w462:dbl)  [unwired: 9 in]
        n156 = call "DriveStraight.vi"("Sensitivity"=0.05, "Range"=0.25, "Motor Speed"=-1.0, "Target"=w462, "Yaw"=w463) -> ("Right"=w471:dbl, "Left"=w472:dbl)  [unwired: 5 in]
        n157 = disable-structure shown="Enabled" {
          disable-tunnel: w472 -> [w494 w519]
          disable-tunnel: w471 -> [w493 w518]
          disable-tunnel: [w490 w519] -> w470
          disable-tunnel: [w489 w518] -> w469
          disable-tunnel: w465 -> [w488 _]
          disable-tunnel: w464 -> [w487 _]
          disable-tunnel: w463 -> [w486 _]
          disable-tunnel: w462 -> [w485 _]
          disable-tunnel: w459 -> [w484 w517]
          disable-tunnel: [w483 w516] -> w458
          frame Disabled {
            n158 = call "DefenseCrosser.vi"("FirstTime?"=w484, "Wait Time"=1.0, "Roll"=w487, "Pitch"=w488, "RightIn"=w493, "LeftIn"=w494) -> ("Complete?"=w480:bool, "RightOut"=w491:dbl, "LeftOut"=w492:dbl)  [unwired: 3 in]
            n159 = feedback #5(FALSE) -> (w478:bool)
            n160 = Select(t=TRUE, s=w480, f=w478) -> (s? t:f=w475:bool)
            n161 = feedback-in #5(w475) -> ()
            n162 = case shown="True" w475 {
              selector: w475 -> [_ w502]
              tunnel: [FALSE w500] -> w481
              frame False {
              }
              frame True {
                n163 = Not(x=w502) -> (.not. x?=w501:bool)
                n164 = feedback-in #6(w501) -> ()
                n165 = feedback #6(TRUE) -> (w500:bool)
              }
            }
            n166 = case shown="True" w475 {
              tunnel: [FALSE ("Completed") w498] -> w482
              tunnel: w481 -> [_ w496]
              frame False {
              }
              frame True {
                n167 = call "Wait Clock.vi"("First Time?"=w496, "Target Time"=1.0) -> ("Completed"=w498:bool)  [unwired: 9 in]
              }
            }
            n168 = case shown="True" w482 {
              tunnel: w492 -> [w505 w514]
              tunnel: w491 -> [w504 w513]
              tunnel: [w505 w512] -> w490
              tunnel: [w504 w511] -> w489
              tunnel: w475 -> [_ w510]
              tunnel: w486 -> [_ w509]
              tunnel: w485 -> [_ w508]
              tunnel: [FALSE ("Complete") w507] -> w483
              frame False {
              }
              frame True {
                n169 = call "Straighten.vi"("Go"=w510, "LockedHeading"=w508, "Yaw"=w509, "RightIn"=w513, "LeftIn"=w514) -> ("Complete"=w507:bool, "RightOut"=w511:dbl, "LeftOut"=w512:dbl)  [unwired: 4 in]
              }
            }
          }
          frame Enabled {
            n170 = call "Wait Clock.vi"("First Time?"=w517, "Target Time"=1.5) -> ("Completed"=w516:bool)  [unwired: 9 in]
          }
        }
        n171 = call "IncrementIndex.vi"("Increment?"=w458, "IndexIn"=w461) -> ("IndexOut"=w460:i32)  [unwired: 9 in]
      }
      frame "Ramparts" {
        # "Ramparts run\nbackwards"
        n172 = call "GyroActions.vi"("navX Device"=w536) -> ("Pitch"=w529:dbl, "Yaw"=w527:dbl, "Roll"=w528:dbl)  [unwired: 6 in, 2 out]
        n173 = Not(x=w523) -> (.not. x?=w535:bool)
        n174 = call "LockedHeading.vi"("LockHeading"=w535, "Heading In"=w527) -> ("LockedHeading"=w526:dbl)  [unwired: 9 in]
        n175 = call "DriveStraight.vi"("Sensitivity"=0.05, "Range"=0.25, "Motor Speed"=-1.0, "Target"=w526, "Yaw"=w527) -> ("Right"=w533:dbl, "Left"=w534:dbl)  [unwired: 5 in]
        n176 = disable-structure shown="Enabled" {
          disable-tunnel: w534 -> [w553 w570]
          disable-tunnel: w533 -> [w552 w569]
          disable-tunnel: w529 -> [w549 _]
          disable-tunnel: w528 -> [w548 _]
          disable-tunnel: w527 -> [w547 _]
          disable-tunnel: w526 -> [w546 _]
          disable-tunnel: w523 -> [w545 w573]
          disable-tunnel: [w544 w572] -> w522
          disable-tunnel: [w539 w569] -> w520
          disable-tunnel: [w538 w570] -> w521
          frame Disabled {
            n177 = call "DefenseCrosser.vi"("FirstTime?"=w545, "Wait Time"=2.0, "Roll"=w548, "Pitch"=w549, "RightIn"=w552, "LeftIn"=w553) -> ("Complete?"=w541:bool, "RightOut"=w550:dbl, "LeftOut"=w551:dbl)  [unwired: 3 in]
            n178 = case shown="True" w541 {
              selector: w541 -> [_ w557]
              tunnel: [FALSE w555] -> w540
              frame False {
              }
              frame True {
                n179 = Not(x=w557) -> (.not. x?=w556:bool)
                n180 = feedback-in #7(w556) -> ()
                n181 = feedback #7(TRUE) -> (w555:bool)
              }
            }
            n182 = call "Wait Clock.vi"("First Time?"=w540, "Target Time"=1.0) -> ("Completed"=w543:bool)  [unwired: 9 in]
            n183 = case shown="False" w543 {
              tunnel: w551 -> [_ w568]
              tunnel: w550 -> [_ w567]
              tunnel: [w560 w566] -> w538
              tunnel: [w560 w565] -> w539
              tunnel: w541 -> [_ w564]
              tunnel: w547 -> [_ w563]
              tunnel: w546 -> [_ w562]
              tunnel: [FALSE ("Complete") w561] -> w544
              frame False {
                w560 = 0.0 ("LeftOut")
              }
              frame True {
                n184 = call "Straighten.vi"("Go"=w564, "LockedHeading"=w562, "Yaw"=w563, "RightIn"=w567, "LeftIn"=w568) -> ("Complete"=w561:bool, "RightOut"=w565:dbl, "LeftOut"=w566:dbl)  [unwired: 4 in]
              }
            }
          }
          frame Enabled {
            n185 = call "Wait Clock.vi"("First Time?"=w573, "Target Time"=2.2) -> ("Completed"=w572:bool)  [unwired: 9 in]
          }
        }
        n186 = call "IncrementIndex.vi"("Increment?"=w522, "IndexIn"=w525) -> ("IndexOut"=w524:i32)  [unwired: 9 in]
      }
      frame "Cheval de Frise" {
        n187 = feedback #8() -> (w577:bool)  [unwired: 1 in]
        n188 = case shown="True" w574 {
          tunnel: [w592 w617] -> w582
          tunnel: [w591 w614] -> w581
          tunnel: w580 -> [w601 _]
          tunnel: [w585 w610] -> w579
          tunnel: [FALSE TRUE] -> w578
          tunnel: w577 -> [w586 _]
          tunnel: w576 -> [w583 w615]
          tunnel: [w584 w615] -> w575
          frame False {
            n189 = call "GyroActions.vi"("navX Device"=w601) -> ("Pitch"=w600:dbl, "Yaw"=w590:dbl, "Roll"=w599:dbl)  [unwired: 6 in, 2 out]
            n190 = Not(x=w586) -> (.not. x?=w587:bool)
            n191 = call "LockedHeading.vi"("LockHeading"=w587, "Heading In"=w590) -> ("LockedHeading"=w589:dbl)  [unwired: 9 in]
            n192 = call "DriveStraight.vi"("Sensitivity"=0.05, "Range"=0.25, "Motor Speed"=-1.0, "Target"=w589, "Yaw"=w590) -> ("Right"=w602:dbl, "Left"=w603:dbl)  [unwired: 5 in]
            n193 = call "DefenseCrosser.vi"("FirstTime?"=w586, "Roll"=w599, "Pitch"=w600, "RightIn"=w602, "LeftIn"=w603) -> ("Complete?"=w593:bool, "RightOut"=w594:dbl, "LeftOut"=w595:dbl)  [unwired: 4 in]
            n194 = call "Straighten.vi"("Go"=w593, "LockedHeading"=w589, "Yaw"=w590, "RightIn"=w594, "LeftIn"=w595) -> ("Complete"=w585:bool, "RightOut"=w591:dbl, "LeftOut"=w592:dbl)  [unwired: 4 in]
            n195 = call "IncrementIndex.vi"("Increment?"=w585, "IndexIn"=w583) -> ("IndexOut"=w584:i32)  [unwired: 9 in]
          }
          frame True {
            w607 = 1070 ("y")
            # "5 in"
            n196 = call "EncoderLeftDrive.vi"() -> ("Position_out"=w609:i32)  [unwired: 11 in]
            n197 = call "EncoderRightDrive.vi"() -> ("Position_out"=w608:i32)  [unwired: 11 in]
            n198 = Greater Or Equal?(x=w609, y=w607) -> (x >= y?=w605:bool)
            n199 = Greater Or Equal?(x=w608, y=w607) -> (x >= y?=w604:bool)
            n200 = Or(x=w605, y=w604) -> (x .or. y?=w606:bool)
            n201 = feedback #9(TRUE) -> (w611:bool)
            n202 = case shown="False" w606 {
              selector: w606 -> [w621 _]
              tunnel: [w626 w638] -> w617
              tunnel: [w625 w638] -> w614
              tunnel: [w620 TRUE ("f")] -> w613
              tunnel: w611 -> [w622 w634]
              tunnel: [TRUE ("Completed") w630] -> w610
              frame False {
                n203 = Select(t=w621, s=w622, f=FALSE) -> (s? t:f=w620:bool)
                n204 = call "GyroActions.vi"() -> ("Yaw"=w623:dbl)  [unwired: 7 in, 4 out]
                n205 = call "LockedHeading.vi"("LockHeading"=w620, "Heading In"=w623) -> ("LockedHeading"=w624:dbl)  [unwired: 9 in]
                n206 = call "DriveStraight.vi"("Sensitivity"=0.05, "Range"=0.25, "Motor Speed"=1.0, "Target"=w624, "Yaw"=w623) -> ("Right"=w625:dbl, "Left"=w626:dbl)  [unwired: 5 in]
              }
              frame True {
                w637 = FALSE
                w638 = 0.0
                n207 = Not(x=w634) -> (.not. x?=w633:bool)
                n208 = call "2Slnd.vi"("AllUp"=w637, "AllDown"=TRUE, "MostUp"=w637, "MostDown"=w637) -> ()  [unwired: 8 in]
                n209 = call "Wait Clock.vi"("First Time?"=w633, "Target Time"=0.5) -> ("Completed"=w631:bool)  [unwired: 9 in]
                n210 = Not(x=w631) -> (.not. x?=w630:bool)
              }
            }
            n211 = feedback-in #9(w613) -> ()
          }
        }
        n212 = feedback-in #8(w578) -> ()
      }
      frame "Portcullis" {
        w649 = FALSE
        n213 = call "Wait Clock.vi"("First Time?"=w647, "Target Time"=0.5) -> ("Completed"=w646:bool)  [unwired: 9 in]
        n214 = call "2Slnd.vi"("AllUp"=w649, "AllDown"=TRUE, "MostUp"=w649, "MostDown"=w649) -> ()  [unwired: 8 in]
        n215 = feedback #10() -> (w639:bool)  [unwired: 1 in]
        n216 = case shown="True" w646 {
          tunnel: [w654 w663] -> w645
          tunnel: [w654 w664] -> w644
          tunnel: w643 -> [w653 w658]
          tunnel: [w653 w657] -> w642
          tunnel: [FALSE w656] -> w641
          tunnel: [FALSE TRUE] -> w640
          tunnel: w639 -> [_ w661]
          frame False {
            w654 = 0.0
          }
          frame True {
            w669 = 19089
            # "89.2 in"
            n217 = call "GyroActions.vi"() -> ("Yaw"=w655:dbl)  [unwired: 7 in, 4 out]
            n218 = call "EncoderLeftDrive.vi"() -> ("Position_out"=w671:i32)  [unwired: 11 in]
            n219 = call "EncoderRightDrive.vi"() -> ("Position_out"=w670:i32)  [unwired: 11 in]
            n220 = call "LockedHeading.vi"("LockHeading"=w661, "Heading In"=w655) -> ("LockedHeading"=w668:dbl)  [unwired: 9 in]
            n221 = Greater Or Equal?(x=w671, y=w669) -> (x >= y?=w659:bool)
            n222 = Greater Or Equal?(x=w670, y=w669) -> (x >= y?=w660:bool)
            n223 = Or(x=w659, y=w660) -> (x .or. y?=w656:bool)
            n224 = call "DriveStraight.vi"("Sensitivity"=0.05, "Range"=0.5, "Motor Speed"=1.0, "Target"=w668, "Yaw"=w655) -> ("Right"=w664:dbl, "Left"=w663:dbl)  [unwired: 5 in]
            n225 = call "IncrementIndex.vi"("Increment?"=w656, "IndexIn"=w658) -> ("IndexOut"=w657:i32)  [unwired: 9 in]
          }
        }
        n226 = feedback-in #10(w640) -> ()
      }
    }
    n227 = call <vilib>:"WPI_RobotDriveTankDrive.vi"("Right axis value"=w76, "Left axis value"=w75, "RobotDriveDevRef"=w74) -> ()  [unwired: 6 in, 3 out]
    n228 = call-poly <vilib>:"NT Write Value.vi"("Boolean"=w64, "Name"="EXIT") -> ()  [unwired: 9 in, 1 out]
  }
